vi "SHA_calc_appendsU64.vi"(11 "String length":i32) -> (1 "Second last chunk":string, 2 "Last Chunk":string, 3 "Number of chunks":i32, 5 "Double appends":bool)   [LabVIEW 2012, in "Encryption.lvlib"]
doc: "Calculates the appendices for the last chunks (64-bit).\n\n(c) Ton Plomp, 2011\nTHIS SOFTWARE IS PROVIDED AS IS, AND ANY WARRANTY IS REJECTED"
uses:
  Encryption.lvlib
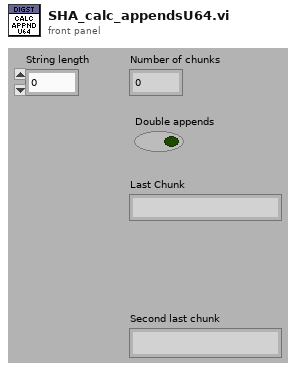
[diagram p1: front panel]
types:
  T1 = enum16{"big-endian, network order", "native, host order", "little-endian"}
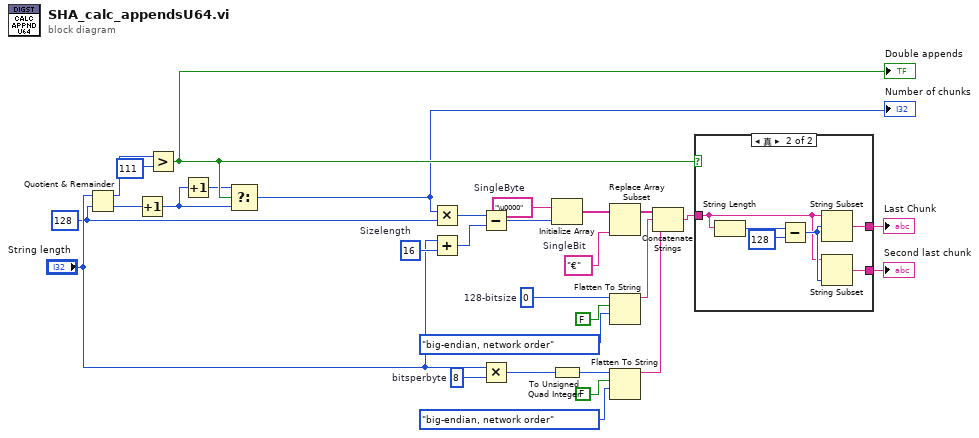
[diagram p0: block diagram]
diagram:
  w3 = u64 0  # 128-bitsize
  w18 = 16  # Sizelength
  w7 = "\u0000"  # SingleByte
  w6 = 8  # bitsperbyte
  w15 = 128 ("y")
  w12 = "€"  # SingleBit
  n1 = Quotient & Remainder(x="String length", y=w15) -> (x-y*floor(x/y)=w23:i32, floor(x/y)=w20:i32)
  n2 = Increment(x=w20) -> (x+1=w25:i32)
  n3 = Greater?(x=w23, y=111) -> (0:w27:bool)
  "Double appends" <- w27
  n4 = Increment(x=w25) -> (x+1=w24:i32)
  n5 = Select(t=w24, s=w27, f=w25) -> (s? t:f=w26:i32)
  "Number of chunks" <- w26
  n6 = Multiply(x=w26, y=w15) -> (x*y=w21:i32)
  n7 = Add(x="String length", y=w18) -> (x+y=w16:i32)
  n8 = Subtract(x=w21, y=w16) -> (x-y=w19:i32)
  n9 = Multiply(x="String length", y=w6) -> (x*y=w8:i32)
  n10 = Initialize Array(w7, w19) -> (w13:string[])
  n11 = To Unsigned Quad Integer(1:w8) -> (0:w9:u64)
  n12 = Replace Array Subset(array=w13, new element=w12) -> (w14:string[])  [unwired: 1 in]
  n13 = Flatten To String(anything=w3, prepend array or string size? (T)=FALSE, byte order (0:big-endian, network order)=T1."big-endian, network order") -> (data string=w2:string)  [unwired: 1 in, 2 out]
  n14 = Flatten To String(anything=w9, prepend array or string size? (T)=FALSE, byte order (0:big-endian, network order)=T1."big-endian, network order") -> (data string=w1:string)  [unwired: 1 in, 2 out]
  n15 = Concatenate Strings(w14, w2, w1) -> (w28:string)
  n16 = case shown="真" w27 {
    tunnel: w28 -> [w31 w32]
    tunnel: [w31 w37] -> w30
    tunnel: [_ w36] -> w29
    frame False {
    }
    frame True {
      n17 = String Length(string=w32) -> (length=w35:i32)
      n18 = Subtract(x=w35, y=128) -> (x-y=w33:i32)
      n19 = String Subset(string=w32, offset (0)=w33) -> (substring=w37:string)  [unwired: 1 in]
      n20 = String Subset(string=w32, length (rest)=w33) -> (substring=w36:string)  [unwired: 1 in]
    }
  }
  "Last Chunk" <- w30
  "Second last chunk" <- w29
